vi "VPA QC Parse String.vi"(10 "Strings In":string[][](array[string]), 11 "Max Line Length":i32=80) -> (2 "Strings Out":string[][](array[string]))   [LabVIEW 2013]
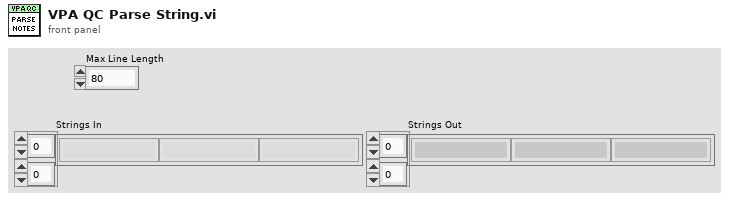
[diagram p1: front panel]
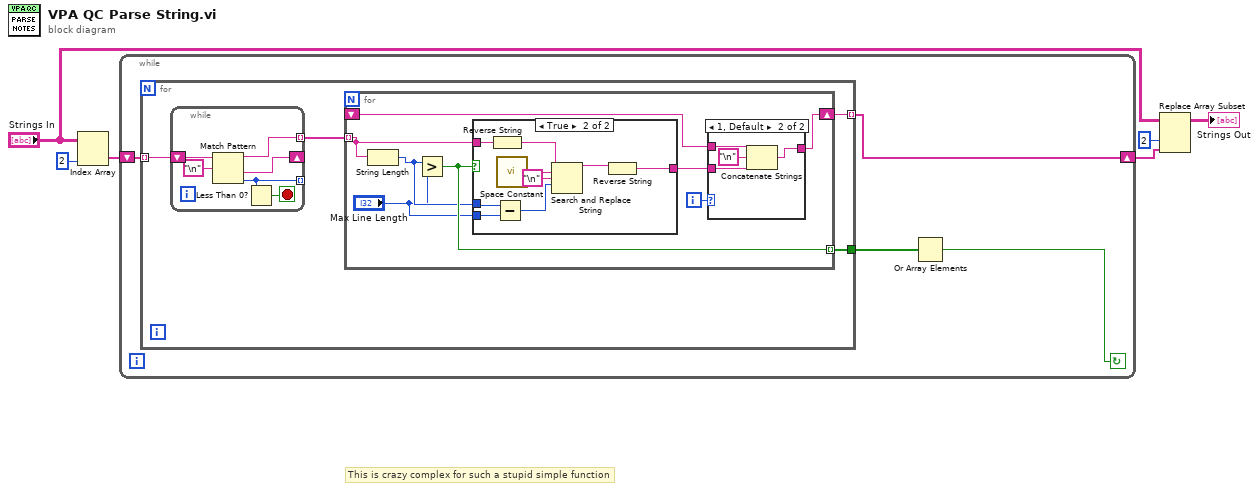
[diagram p0: block diagram]
diagram:
  # "This is crazy complex for such a stupid simple function"
  n1 = Index Array(array="Strings In", index (col)=2 ("disabled index (col)")) -> (element=w5:string[])  [unwired: 1 in]
  n2 = while {
    shift-right: [w9] -> w2
    shift-left: w5 -> [w10]
    stop <- w7 continue-if-true
    n3 = for {
      tunnel: w10 -> [w12] mode=indexing
      tunnel: [w14] -> w9 mode=indexing
      tunnel: [w13] -> w8
      n4 = while {
        tunnel: [w43] -> w11 mode=indexing
        tunnel: [w41] -> _ mode=indexing
        shift-right: [w38] -> _
        shift-left: w12 -> [w39]
        stop <- w42 stop-if-true
        n5 = Match Pattern(string=w39, regular expression="\n") -> (before substring=w43:string, after substring=w38:string, offset past match=w41:i32)  [unwired: 1 in, 1 out]
        n6 = Less Than 0?(x=w41) -> (x < 0?=w42:bool)
      }
      n7 = for {
        tunnel: w11 -> [w21] mode=indexing
        tunnel: [w22] -> w13 mode=indexing
        shift-right: [w18] -> w14
        shift-left: _ -> [w17]
        i -> [w20]
        n8 = String Length(string=w21) -> (length=w16:i32)
        n9 = Greater?(x=w16, y="Max Line Length") -> (0:w22:bool)
        n10 = case shown="True" w22 {
          tunnel: w21 -> [w28 w37]
          tunnel: [w28 w33] -> w19
          tunnel: w16 -> [_ w30]
          tunnel: "Max Line Length" -> [_ w31]
          frame False {
          }
          frame True {
            n11 = Reverse String(1:w37) -> (0:w36:string)
            n12 = Subtract(x=w30, y=w31) -> (x-y=w29:i32)
            n13 = call <vilib>:"Space Constant.vi"() -> ("String"=w35:string)
            n14 = Search and Replace String(input string=w36, search string=w35, replace string="\n" ("replace string (\"\")"), offset=w29) -> (result string=w34:string)  [unwired: 4 in, 3 out]
            n15 = Reverse String(1:w34) -> (0:w33:string)
          }
        }
        n16 = case shown="1, Default" w20 {
          tunnel: w19 -> [w23 w25]
          tunnel: [w23 w24] -> w18
          tunnel: w17 -> [_ w27]
          frame 0 {
          }
          frame 1, Default {
            n17 = Concatenate Strings(w27, "\n" ("string"), w25) -> (w24:string)
          }
        }
      }
    }
    n18 = Or Array Elements(Boolean array=w8) -> (logical OR=w7:bool)
  }
  n19 = Replace Array Subset(array="Strings In", new element=w2, index (col)=2 ("disabled index (col)")) -> (→"Strings Out":string[][])  [unwired: 1 in]
